vi "LVH5AwriteWDTAttrs.vi"(8 "error in (no error)":errorcluster, 9 "dt":dbl, 10 "t0":timestamp, 11 "Waveform Dataset Ref":T1) -> (0 "error out":errorcluster, 3 "Waveform Dataset Ref out":T1)   [LabVIEW 2017]
uses:
  <vilib>/UPVI/lvhdf5/library.llb/HDF5 Ref.ctl
  <vilib>/UPVI/lvhdf5/attribute.llb/LVH5A Operation.ctl
panel:
  # "LVHDF5 Toolkit\nCopyright (c) 2005-2013 by Jason D. Sommerville\nCopyright (c) 2014 by UPVI, LLC.\n\nThis use and distribution of this file is governed by the terms found in \nLICENSE.txt distributed with this toolkit and installed at\n <user.lib>\\_lvhdf5\\LICENSE.txt"
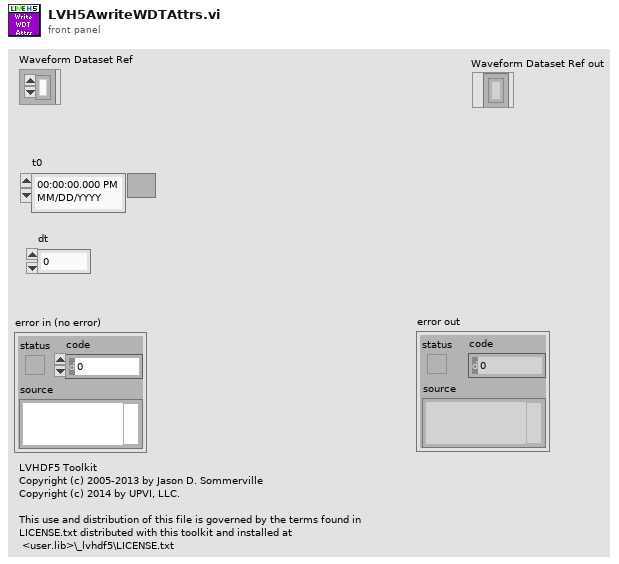
[diagram p1: front panel]
types:
  T1 = typedef "HDF5 Ref.ctl" = refnum<k1>
  T2 = typedef "LVH5A Operation.ctl" = enum16{"open", "replace", "create", "open or create", "create or replace", "create or replace with confirmation"}
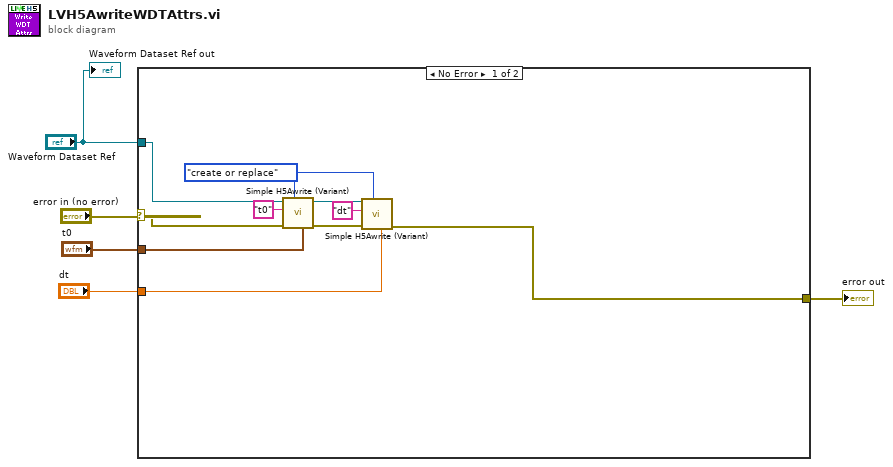
[diagram p0: block diagram]
diagram:
  n1 = case shown="No Error" "error in (no error)" {
    selector: "error in (no error)" -> [w7 w16]
    tunnel: "Waveform Dataset Ref" -> [w14 _]
    tunnel: [w6 w16] -> w3
    tunnel: "t0" -> [w15 _]
    tunnel: "dt" -> [w12 _]
    frame No Error {
      w11 = LVH5A_Operation."create or replace" ("operation (open or create)")
      n2 = call <vilib>:"Simple H5Awrite (Variant).vi"("Value"=w15, "operation (open or create)"=w11, "error in (no error)"=w7, "Name"="t0", "HDF5 Ref"=w14) -> ("error out"=w8:errorcluster, "HDF5 Ref out"=w10:T1)  [unwired: 3 in]
      n3 = call <vilib>:"Simple H5Awrite (Variant).vi"("Value"=w12, "operation (open or create)"=w11, "error in (no error)"=w8, "Name"="dt", "HDF5 Ref"=w10) -> ("error out"=w6:errorcluster)  [unwired: 3 in, 1 out]
    }
    frame Error {
    }
  }
  "error out" <- w3
  "Waveform Dataset Ref out" <- "Waveform Dataset Ref"
